vi "Difference.vi"(7 "error in (no error)":errorcluster, 8 "Compare to this JSON Object":string="{}", 10 "JSON Object":string="{}") -> (0 "error out":errorcluster, 3 "<JSON>":string caption="<JSON>Changes")   [LabVIEW 2015, in "JSONtext.lvlib"]
doc: "Compares (\"Diffs\") a JSON Object to another JSON Object.\n\nReturns a reduced-size Object that includes only changed elements."
uses:
  JSONtext.lvlib
  support/Format JSON Object.vi
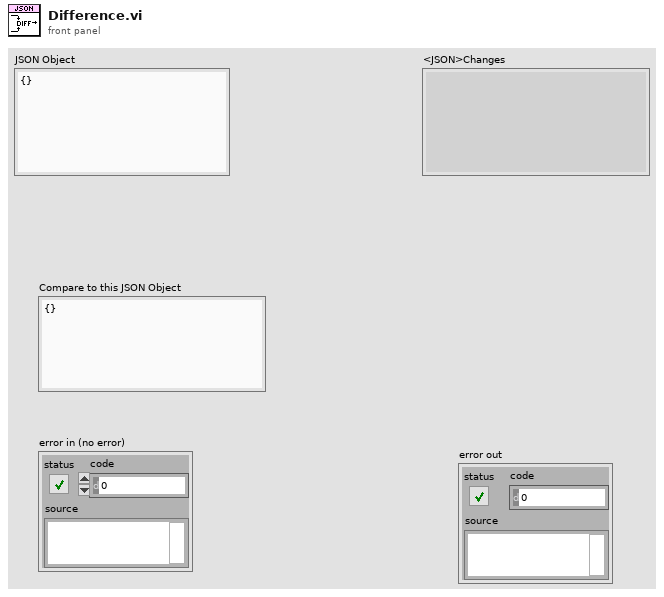
[diagram p1: front panel]
types:
  T1 = typedef "JSON Value Type.ctl" = enum16{"Not a JSON Value", "JSON Object", "JSON Array", "String", "Number", "true", "false", "null"}
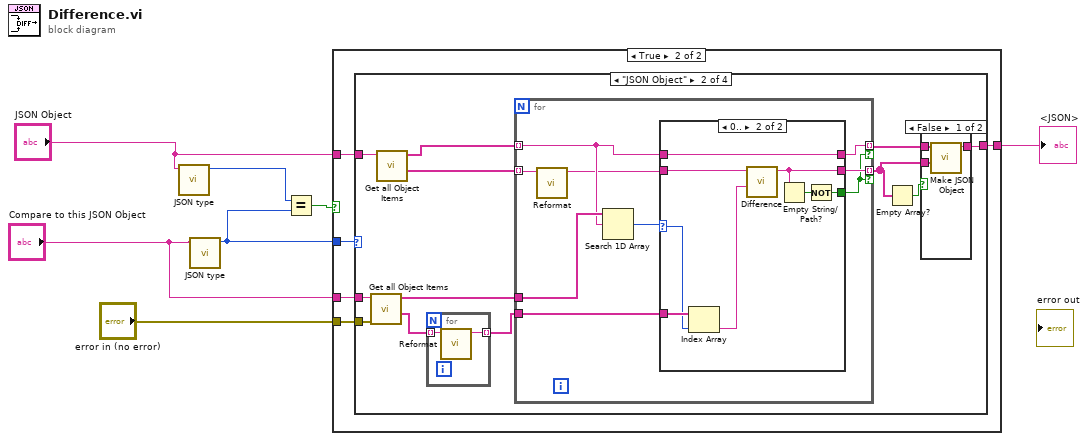
[diagram p0: block diagram]
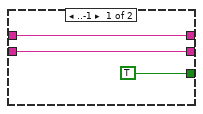
[diagram p5: hidden frame]
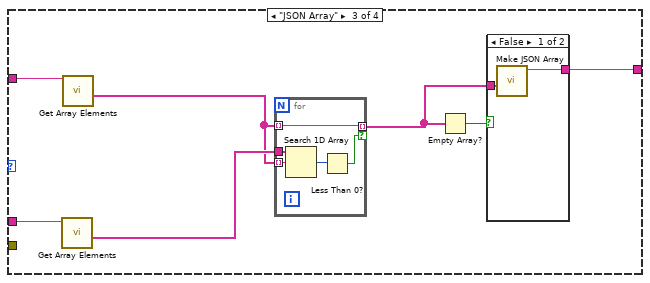
[diagram p6: hidden frame]
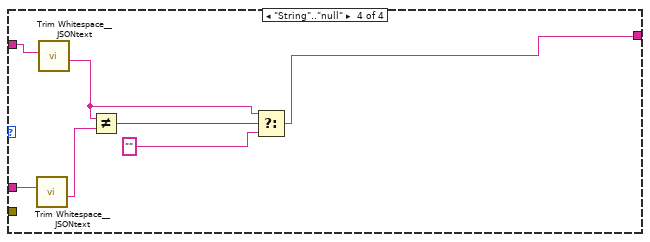
[diagram p8: hidden frame]
diagram:
  n1 = call "JSON type.vi"("JSON"="JSON Object") -> ("JSON Value Type"=w3:T1)  [unwired: 9 in, 1 out]
  n2 = call "JSON type.vi"("JSON"="Compare to this JSON Object") -> ("JSON Value Type"=w1:T1)  [unwired: 9 in, 1 out]
  n3 = Equal?(x=w3, y=w1) -> (x = y?=w2:bool)
  n4 = case shown="True" w2 {
    tunnel: "error in (no error)" -> [_ w13]
    tunnel: [w8 w12] -> w6
    tunnel: "JSON Object" -> [w8 w11]
    tunnel: "Compare to this JSON Object" -> [_ w10]
    tunnel: w1 -> [_ w9]
    frame False {
    }
    frame True {
      n5 = case shown="\"JSON Object\"" w9 {
        tunnel: w13 -> [_ w26 _ _]
        tunnel: [w14 w21 w54 w66] -> w12
        tunnel: w11 -> [w14 w20 w58 w72]
        tunnel: w10 -> [_ w19 w57 w71]
        frame "Not a JSON Value", Default {
        }
        frame "JSON Object" {
          n6 = call "Get all Object Items.vi"("error in (no error)"=w26, "JSON"=w19) -> ("<JSON>"=w16:string[], "Names"=w24:string[])  [unwired: 6 in, 2 out]
          n7 = call "Get all Object Items.vi"("JSON"=w20) -> ("<JSON>"=w23:string[], "Names"=w25:string[])  [unwired: 7 in, 2 out]
          n8 = for {
            tunnel: w16 -> [w28] mode=indexing
            tunnel: [w27] -> w15 mode=indexing
            n9 = call "Reformat.vi"("Input String"=w28) -> ("<JSON>First JSON Value"=w27:string)  [unwired: 6 in, 3 out]
          }
          n10 = for {
            tunnel: w25 -> [w34] mode=indexing
            tunnel: w24 -> [w40]
            tunnel: w23 -> [w33] mode=indexing
            tunnel: [w38] -> w22 mode=indexing if=w36
            tunnel: [w37] -> w18 mode=indexing if=w36
            tunnel: w15 -> [w35]
            n11 = call "Reformat.vi"("Input String"=w33) -> ("<JSON>First JSON Value"=w32:string)  [unwired: 6 in, 3 out]
            n12 = Search 1D Array(1D array=w40, element=w34) -> (index of element=w39:i32)  [unwired: 1 in]
            n13 = case shown="0.." w39 {
              selector: w39 -> [_ w50]
              tunnel: w34 -> [w43 w47]
              tunnel: w32 -> [w42 w48]
              tunnel: [w43 w47] -> w38
              tunnel: [w42 w46] -> w37
              tunnel: [TRUE w45] -> w36
              tunnel: w35 -> [_ w51]
              frame ..-1 {
              }
              frame 0.. {
                n14 = Index Array(array=w51, index=w50) -> (element=w49:string)
                n15 = call "Difference.vi"("Compare to this JSON Object"=w49, "JSON Object"=w48) -> ("<JSON>"=w46:string)  [unwired: 7 in, 1 out]
                n16 = Empty String/Path?(string/path=w46) -> (empty?=w44:bool)
                n17 = Not(x=w44) -> (.not. x?=w45:bool)
              }
            }
          }
          n18 = Empty Array?(array=w18) -> (empty?=w17:bool)
          n19 = case shown="False" w17 {
            tunnel: w22 -> [w31 _]
            tunnel: [w30 _] -> w21
            tunnel: w18 -> [w29 _]
            frame False {
              n20 = call "Make JSON Object.vi"("JSON elements"=w29, "Names"=w31) -> ("JSON Object Text out"=w30:string)  [unwired: 8 in, 1 out]
            }
            frame True {
            }
          }
        }
        frame "JSON Array" {
          n21 = call "Get Array Elements.vi"("JSON"=w57) -> ("<JSON>"=w56:string[])  [unwired: 8 in, 2 out]
          n22 = call "Get Array Elements.vi"("JSON"=w58) -> ("<JSON>"=w55:string[])  [unwired: 8 in, 2 out]
          n23 = for {
            tunnel: w56 -> [w65]
            tunnel: w55 -> [w64] mode=indexing
            tunnel: [w63] -> w53 mode=indexing if=w61
            tunnel: w55 -> [w63] mode=indexing
            n24 = Search 1D Array(1D array=w65, element=w64) -> (index of element=w62:i32)  [unwired: 1 in]
            n25 = Less Than 0?(x=w62) -> (x < 0?=w61:bool)
          }
          n26 = Empty Array?(array=w53) -> (empty?=w52:bool)
          n27 = case shown="False" w52 {
            tunnel: [w60 _] -> w54
            tunnel: w53 -> [w59 _]
            frame False {
              n28 = call "Make JSON Array.vi"("Array of JSON Text"=w59) -> ("<JSON>Array"=w60:string)  [unwired: 9 in, 1 out]
            }
            frame True {
            }
          }
        }
        frame "String".."null" {
          n29 = call "Trim Whitespace__JSONtext.vi"("String in"=w71) -> ("String out"=w70:string)  [unwired: 6 in]
          n30 = call "Trim Whitespace__JSONtext.vi"("String in"=w72) -> ("String out"=w67:string)  [unwired: 6 in]
          n31 = Not Equal?(x=w67, y=w70) -> (x != y?=w69:bool)
          n32 = Select(t=w67, s=w69, f="") -> (s? t:f=w66:string)
        }
      }
    }
  }
  "<JSON>" <- w6
